vi "Queue Reference (library variable).vi"() -> ()   [LabVIEW 2016, in "Error Manager.lvlib" / "MHL Queue.lvclass"]
uses:
  MHL Queue.lvclass
  Command (enum).ctl
  Message (cluster).ctl
panel:
  in  "Queue Reference":refnum<queue>
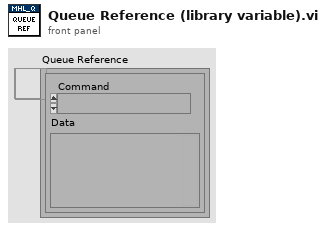
[diagram p1: front panel]
diagram:
